vi "TestKCubeConnection.vi"() -> ()   [LabVIEW 2020]
uses:
  C:/GEECS/Developers Version/source/Device Drivers/KinesisCube/Thorlabs.MotionControl.KCube.PiezoCLI.dll
  Thorlabs.MotionControl.KCube.PiezoCLI.dll
  C:/GEECS/Developers Version/source/Device Drivers/KinesisCube/Thorlabs.MotionControl.Controls.dll
  Thorlabs.MotionControl.Controls.dll
panel:
  out "CloseDevice":bool
  out "KCube":refnum<k24>
  out "CreateDevice":bool
  in  "state":i32(ring) items=["Disconnected", "Connecting", "PreConnecting", "Connected"]
  in  "delayTime":i32
  out "Device":refnum<k24>
  out "IsConnected":bool
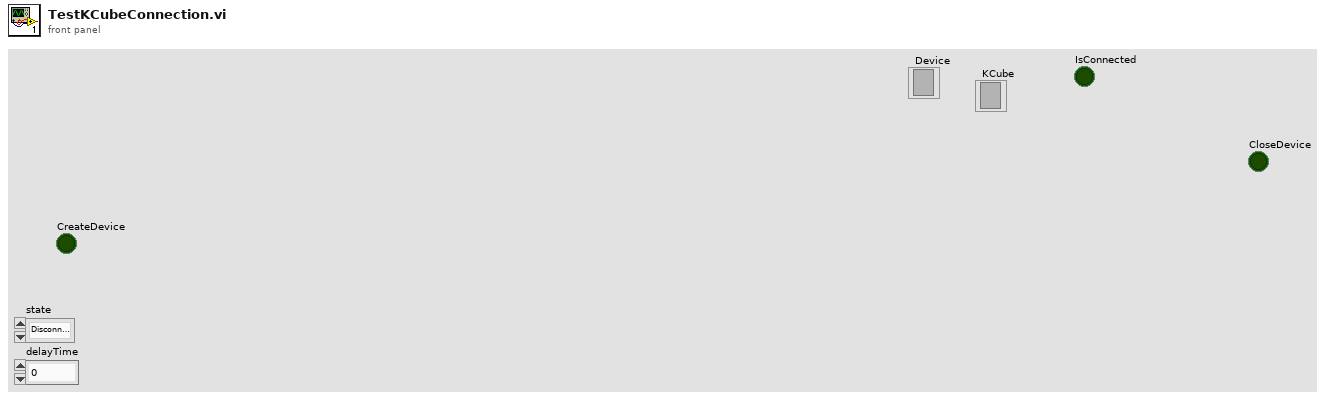
[diagram p1: front panel]
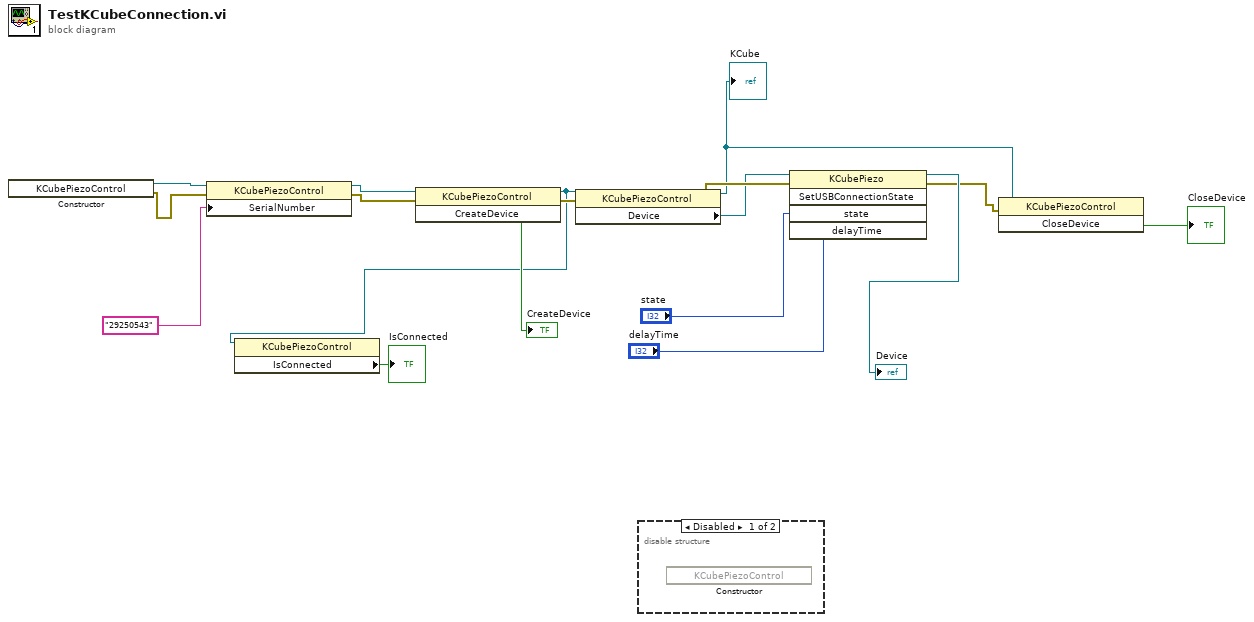
[diagram p0: block diagram]
diagram:
  n1 = constructor class="KCubePiezoControl"() -> (reference out=w7:refnum<k24>, error out=w6:errorcluster)  [unwired: 3 in, 1 out]
  n2 = property class="KCubePiezoControl"(reference=w7, error in=w6, "SerialNumber"="29250543") -> (reference out=w10:refnum<k24>, error out=w17:errorcluster)
  n3 = invoke class="KCubePiezoControl" method="CreateDevice"(reference=w10, error in=w17) -> (reference out=w8:refnum<k24>, error out=w16:errorcluster, "CreateDevice"=→"CreateDevice":bool)  [unwired: 1 in]
  n4 = property class="KCubePiezoControl"(reference=w8) -> ("IsConnected"=→"IsConnected":bool)  [unwired: 1 in, 2 out]
  n5 = property class="KCubePiezoControl"(reference=w8, error in=w16) -> (reference out=w2:refnum<k24>, error out=w15:errorcluster, "Device"=w11:refnum<k24>)
  "KCube" <- w2
  n6 = disable-structure shown="Disabled" {
    frame Disabled {
      n7 = constructor class="KCubePiezoControl"() -> ()  [unwired: 3 in, 3 out]
    }
    frame Enabled {
    }
  }
  n8 = invoke class="KCubePiezo" method="SetUSBConnectionState"(reference=w11, error in=w15, "state"="state", "delayTime"="delayTime") -> (reference out=→"Device":refnum<k24>, error out=w1:errorcluster)  [unwired: 1 in, 3 out]
  n9 = invoke class="KCubePiezoControl" method="CloseDevice"(reference=w2, error in=w1) -> ("CloseDevice"=→"CloseDevice":bool)  [unwired: 1 in, 2 out]
